vi "Phoenix2.vi"() -> ()   [LabVIEW 2018]
uses:
  Game_class/Game.lvclass
panel:
  in  "Game in":refnum<class "Game.lvclass">
  out "Game out":refnum<class "Game.lvclass">
  in  "Game":refnum<class "Game.lvclass">
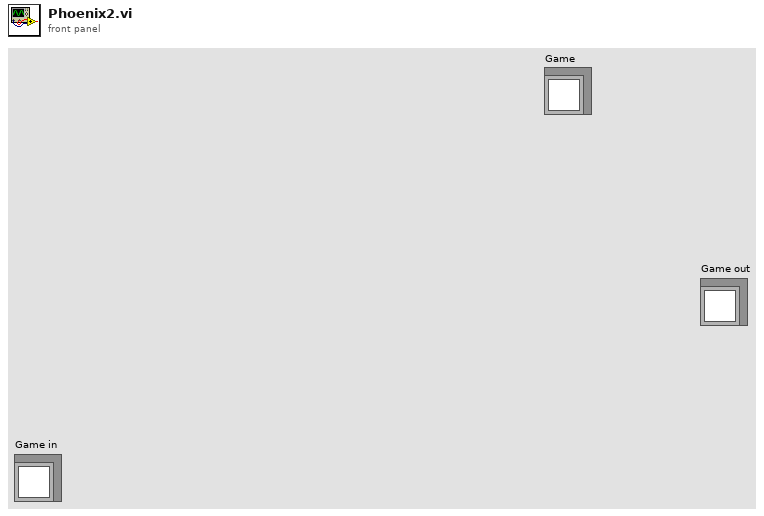
[diagram p1: front panel]
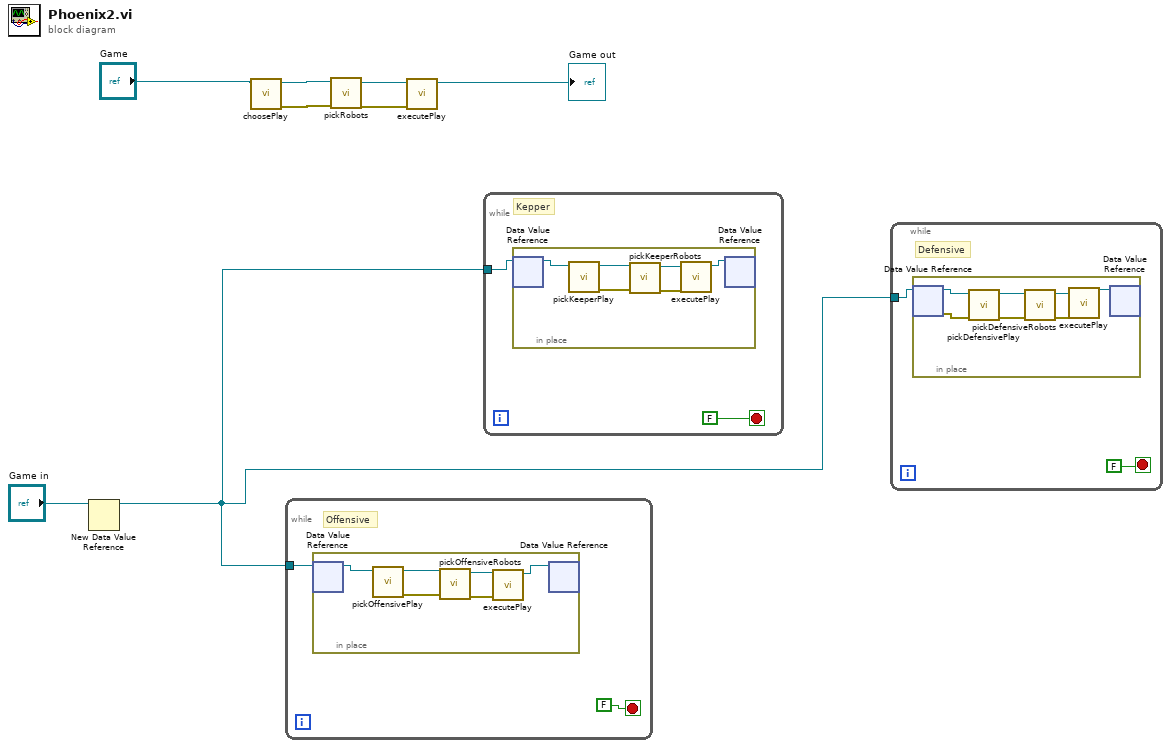
[diagram p0: block diagram]
diagram:
  n1 = New Data Value Reference(data value="Game in") -> (data value reference=w2:refnum<data-value>)  [unwired: 1 in, 1 out]
  n2 = call-dynamic "choosePlay.vi"("Game in"="Game") -> ("error out"=w7:errorcluster, "Game out"=w8:refnum<class "Game.lvclass">)  [unwired: 9 in]
  n3 = while {
    tunnel: w2 -> [w9]
    stop <- FALSE stop-if-true
    # "Offensive"
    n4 = in-place {
      n5 = in-place-dvr #1(w9) -> (w14:refnum<class "Game.lvclass">)  [unwired: 1 out]
      n6 = call-dynamic "pickOffensivePlay.vi"("Game in"=w14) -> ("error out"=w15:errorcluster, "Game out"=w16:refnum<class "Game.lvclass">)  [unwired: 9 in]
      n7 = call-dynamic "pickOffensiveRobots.vi"("error in (no error)"=w15, "Game in"=w16) -> ("error out"=w12:errorcluster, "Game out"=w13:refnum<class "Game.lvclass">)  [unwired: 8 in]
      n8 = call-dynamic "executePlay.vi"("error in (no error)"=w12, "Game in"=w13) -> ("Game out"=w11:refnum<class "Game.lvclass">)  [unwired: 8 in, 1 out]
      n9 = in-place-dvr #1(w11) -> ()  [unwired: 2 out]
    }
  }
  n10 = call-dynamic "pickRobots.vi"("error in (no error)"=w7, "Game in"=w8) -> ("error out"=w5:errorcluster, "Game out"=w6:refnum<class "Game.lvclass">)  [unwired: 8 in]
  n11 = call-dynamic "executePlay.vi"("error in (no error)"=w5, "Game in"=w6) -> ("Game out"=→"Game out":refnum<class "Game.lvclass">)  [unwired: 8 in, 1 out]
  n12 = while {
    tunnel: w2 -> [w17]
    stop <- FALSE stop-if-true
    # "Kepper"
    n13 = in-place {
      n14 = in-place-dvr #2(w17) -> (w22:refnum<class "Game.lvclass">)  [unwired: 1 out]
      n15 = call-dynamic "pickKeeperPlay.vi"("Game in"=w22) -> ("error out"=w23:errorcluster, "Game out"=w24:refnum<class "Game.lvclass">)  [unwired: 9 in]
      n16 = call-dynamic "pickKeeperRobots.vi"("error in (no error)"=w23, "Game in"=w24) -> ("error out"=w20:errorcluster, "Game out"=w21:refnum<class "Game.lvclass">)  [unwired: 8 in]
      n17 = call-dynamic "executePlay.vi"("error in (no error)"=w20, "Game in"=w21) -> ("Game out"=w19:refnum<class "Game.lvclass">)  [unwired: 8 in, 1 out]
      n18 = in-place-dvr #2(w19) -> ()  [unwired: 2 out]
    }
  }
  n19 = while {
    tunnel: w2 -> [w25]
    stop <- FALSE stop-if-true
    # "Defensive"
    n20 = in-place {
      n21 = in-place-dvr #3(w25) -> (w31:refnum<class "Game.lvclass">, w30:errorcluster)
      n22 = call-dynamic "pickDefensivePlay.vi"("error in (no error)"=w30, "Game in"=w31) -> ("error out"=w32:errorcluster, "Game out"=w33:refnum<class "Game.lvclass">)  [unwired: 8 in]
      n23 = call-dynamic "pickDefensiveRobots.vi"("error in (no error)"=w32, "Game in"=w33) -> ("error out"=w28:errorcluster, "Game out"=w29:refnum<class "Game.lvclass">)  [unwired: 8 in]
      n24 = call-dynamic "executePlay.vi"("error in (no error)"=w28, "Game in"=w29) -> ("Game out"=w27:refnum<class "Game.lvclass">)  [unwired: 8 in, 1 out]
      n25 = in-place-dvr #3(w27) -> ()  [unwired: 2 out]
    }
  }
